vi "Max_&_Min_Array.vi"(0 "Choose Max & Min Array":T2, 2 "Max & Min Array 1D":i8[](array[numeric])=[1, -1, 2, 100, 10], 3 "Max & Min Array 2D":i8[][](array[numeric])=[[-3, 55, 41], [6, -1, 14], [-3, 2, -70], [-100, 1, 7]]) -> (14 "Max. Value":i8, 15 "Index Max.":i32, 16 "Indexs Max.":T1, 17 "Min. Value":i8, 18 "Index Min.":i32, 19 "Indexs Min.":T1)   [LabVIEW 2018]
uses:
  Controls/1D_2D.ctl
  Controls/Rows_Columns.ctl
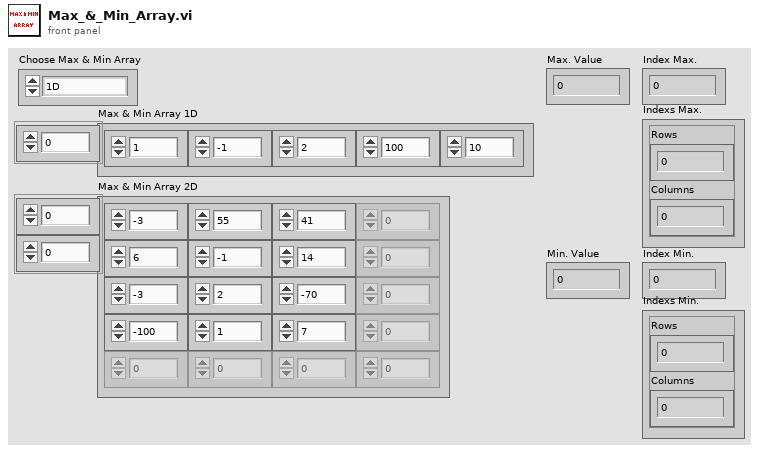
[diagram p1: front panel]
types:
  T1 = typedef "Rows_Columns.ctl" = cluster{"Rows":i32, "Columns":i32}
  T2 = typedef "1D_2D.ctl" = enum16{"1D", "2D"}
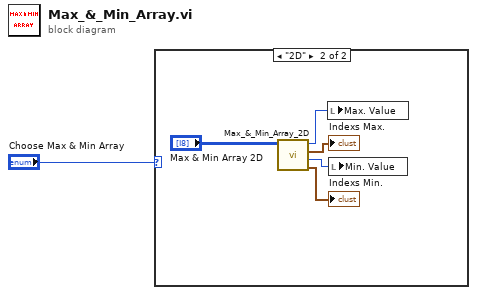
[diagram p0: block diagram]
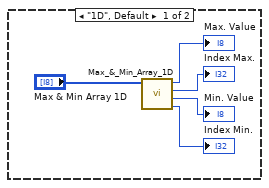
[diagram p2: hidden frame]
diagram:
  n1 = case shown="\"2D\"" "Choose Max & Min Array" {
    frame "1D", Default {
      n2 = call "Max_&_Min_Array_1D.vi"("Max & Min Array 1D"="Max & Min Array 1D") -> ("Index Min."=→"Index Min.":i32, "Min. Value"=→"Min. Value":i8, "Index Max."=→"Index Max.":i32, "Max. Value"=→"Max. Value":i8)  [unwired: 7 in]
    }
    frame "2D" {
      n3 = call "Max_&_Min_Array_2D.vi"("Max & Min Array 2D"="Max & Min Array 2D") -> ("Indexs Min."=→"Indexs Min.":T1, "Min. Value"=w10:i8, "Indexs Max."=→"Indexs Max.":T1, "Max. Value"=w9:i8)  [unwired: 7 in]
      n4 = local write "Max. Value"(w9) -> ()
      n5 = local write "Min. Value"(w10) -> ()
    }
  }
